vi "FindAllChildDotGitFolders.vi"(8 "error in":errorcluster, 11 "Path":path) -> (0 "error out":errorcluster, 2 "Number of git's including parent":i32, 3 "All .git paths from parent":path[](array[path]))   [LabVIEW 2018, in "feGEM DataPacker.lvlib"]
uses:
  feGEM DataPacker.lvlib
  <userlib>/_RADE/MTA-lib/file/file.llb/Strip Path - Traditional__ogtk.vi
panel:
  out "All Folders":path[](array[path])
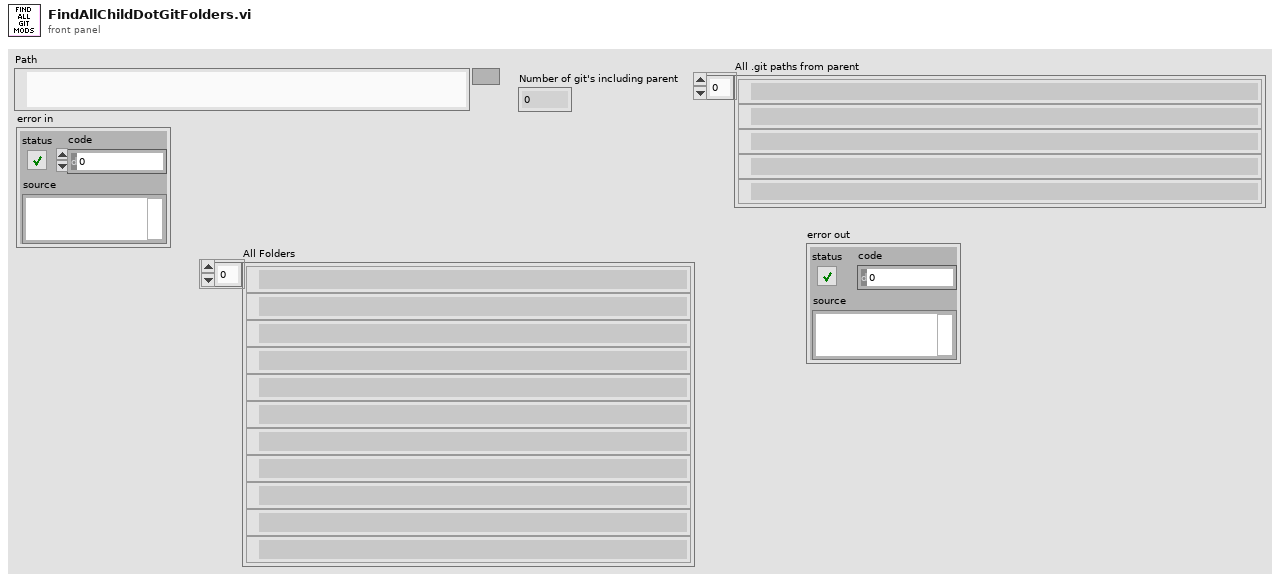
[diagram p1: front panel]
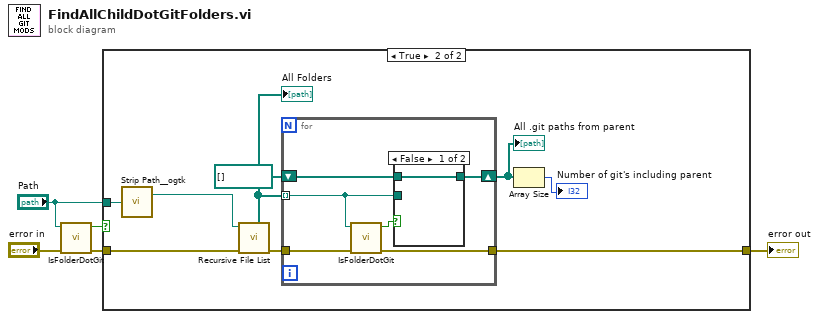
[diagram p0: block diagram]
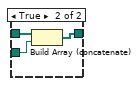
[diagram p3: hidden frame]
diagram:
  n1 = call "IsFolderDotGit.vi"("error in"="error in", "path"="Path") -> ("error out"=w2:errorcluster, "Is .git folder"=w4:bool)  [unwired: 8 in]
  n2 = case shown="True" w4 {
    tunnel: "Path" -> [_ w12]
    tunnel: w2 -> [w6 w11]
    tunnel: [w6 w9] -> w1
    frame False {
    }
    frame True {
      n3 = call-poly <userlib>:"Strip Path__ogtk.vi"("path"=w12) -> ("stripped path"=w8:path)  [unwired: 1 out]
      n4 = call <vilib>:"Recursive File List.vi"("error in (no error)"=w11, "Folder Path"=w8) -> ("error out"=w10:errorcluster, "All Folders"=w15:path[])  [unwired: 5 in, 3 out]
      "All Folders" <- w15
      n5 = for {
        tunnel: w15 -> [w19] mode=indexing
        shift-right: [w21] -> w14
        shift-left: path[] [] -> [w20]
        tunnel: w10 -> [w17]
        tunnel: [w16] -> w9
        n6 = call "IsFolderDotGit.vi"("error in"=w17, "path"=w19) -> ("error out"=w16:errorcluster, "Is .git folder"=w18:bool)  [unwired: 8 in]
        n7 = case shown="False" w18 {
          tunnel: w19 -> [_ w25]
          tunnel: [w22 w24] -> w21
          tunnel: w20 -> [w22 w23]
          frame False {
          }
          frame True {
            n8 = Build Array (concatenate)(w23, w25) -> (w24:path[])
          }
        }
      }
      "All .git paths from parent" <- w14
      n9 = Array Size(array=w14) -> (size(s)=→"Number of git's including parent":i32)
    }
  }
  "error out" <- w1
